vi "LoopSafe.vi"(6 "ModeChange Cluster":T1, 8 "error in (no error)":errorcluster, 11 "ModeCol in":refnum<class "ModeCol.lvclass">) -> (0 "error out":errorcluster, 3 "ModeCol out":refnum<class "ModeCol.lvclass">)   [LabVIEW 2013, in "ModeCol.lvclass"]
doc: "This VI check that there are no ramps between Loop-EndLoop pairs. It should be called only for \"Loop\" or \"EndLoop\" item tags."
uses:
  ModeCol.lvclass
  TypeDefs/ModeChange.ctl
  <vilib>/Utility/miscctls.llb/LVRowAndColumnTypeDef.ctl
  TypeDefs/TableHistory.ctl
  TypeDefs/TableArray.ctl
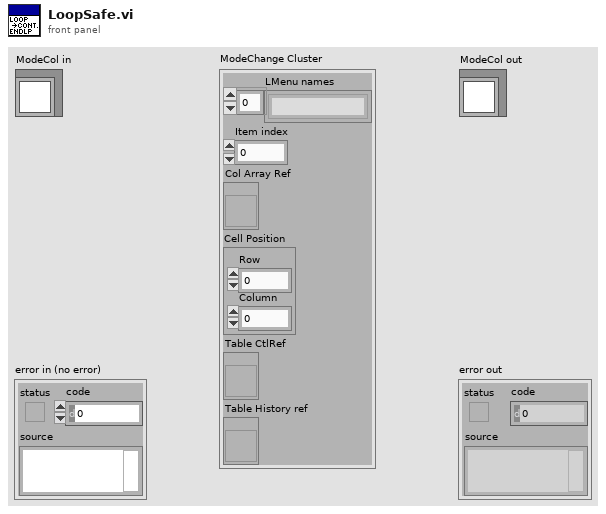
[diagram p1: front panel]
types:
  T1 = typedef "ModeChange.ctl" = cluster{"LMenu names":string[], "Item index":i32, "Col Array Ref":refnum<vi>, "Cell Position":T2, "Table CtlRef":refnum<vi>, "Table History ref":refnum<vi>}
  T2 = typedef "LVRowAndColumnTypeDef.ctl" = cluster{"Row":i32, "Column":i32}
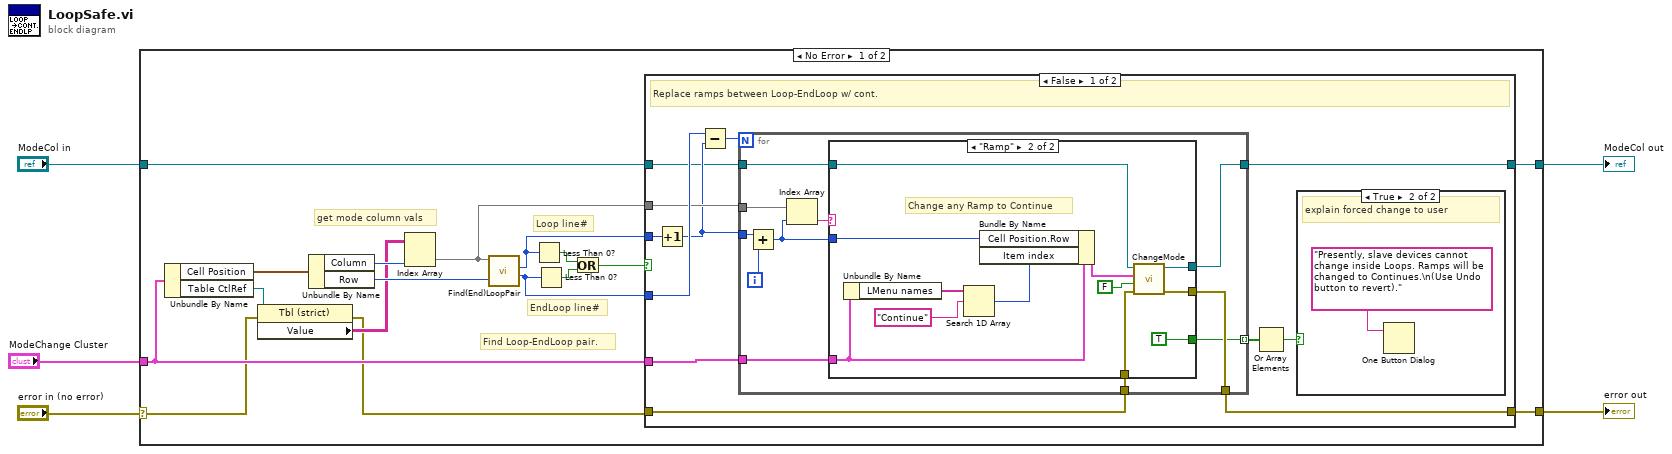
[diagram p0: block diagram]
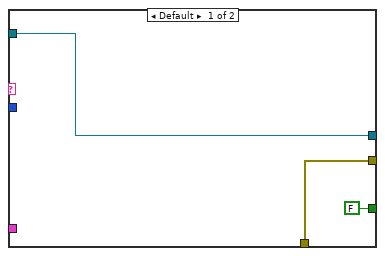
[diagram p3: hidden frame]
diagram:
  n1 = case shown="No Error" "error in (no error)" {
    selector: "error in (no error)" -> [w7 w65]
    tunnel: [w19 w65] -> w4
    tunnel: [w21 w64] -> w2
    tunnel: "ModeCol in" -> [w20 w64]
    tunnel: "ModeChange Cluster" -> [w10 _]
    frame No Error {
      # "Find Loop-EndLoop pair."
      # "EndLoop line#"
      # "Loop line#"
      # "get mode column vals"
      n2 = Unbundle By Name(w10) -> ("Cell Position"=w11:T2, "Table CtlRef"=w9:refnum<vi>)
      n3 = property class="Tbl (strict)"(reference=w9, error in=w7) -> (error out=w6:errorcluster, "Value"=w8:string[][])  [unwired: 1 out]
      n4 = Unbundle By Name(w11) -> ("Column"=w18:i32, "Row"=w22:i32)
      n5 = Index Array(array=w8, index (col)=w18) -> (element=w17:string[])  [unwired: 1 in]
      n6 = call "Find(End)LoopPair.vi"("(End)Loop index"=w22, "Mode Array"=w17) -> ("EndLoop index"=w12:i32, "Loop index"=w13:i32)  [unwired: 8 in]
      n7 = Less Than 0?(x=w13) -> (x < 0?=w15:bool)
      n8 = Less Than 0?(x=w12) -> (x < 0?=w16:bool)
      n9 = Or(x=w15, y=w16) -> (x .or. y?=w14:bool)
      n10 = case shown="False" w14 {
        tunnel: [w25 w63] -> w21
        tunnel: w20 -> [w26 w63]
        tunnel: [w33 w62] -> w19
        tunnel: w6 -> [w34 w62]
        tunnel: w13 -> [w31 _]
        tunnel: w12 -> [w30 _]
        tunnel: w17 -> [w28 _]
        tunnel: w10 -> [w32 _]
        frame False {
          # "Replace ramps between Loop-EndLoop w/ cont."
          n11 = Increment(x=w31) -> (x+1=w27:i32)
          n12 = Subtract(x=w30, y=w27) -> (x-y=w29:i32)
          n13 = for {
            N: w29 -> [_]
            tunnel: w34 -> [w46]
            tunnel: [w45] -> w33
            tunnel: w32 -> [w44]
            tunnel: w28 -> [w43]
            tunnel: w27 -> [w41]
            tunnel: w26 -> [w40]
            tunnel: [w39] -> w25
            tunnel: [w36] -> w24 mode=indexing
            i -> [w42]
            n14 = Add(x=w41, y=w42) -> (x+y=w37:i32)
            n15 = Index Array(array=w43, index=w37) -> (element=w38:string)
            n16 = case shown="\"Ramp\"" w38 {
              tunnel: w46 -> [w48 w59]
              tunnel: [w48 w60] -> w45
              tunnel: w44 -> [_ w55]
              tunnel: w40 -> [w49 w58]
              tunnel: [w49 w61] -> w39
              tunnel: w37 -> [_ w56]
              tunnel: [FALSE TRUE] -> w36
              frame Default {
              }
              frame "Ramp" {
                # "Change any Ramp to Continue"
                n17 = Unbundle By Name(w55) -> ("LMenu names"=w54:string[])
                n18 = Search 1D Array(1D array=w54, element="Continue") -> (index of element=w52:i32)  [unwired: 1 in]
                n19 = Bundle By Name(cluster=w55, "Cell Position.Row"=w56, "Item index"=w52) -> (w57:T1)
                n20 = call-dynamic "ChangeMode.vi"("error in (no error)"=w59, "Save to TblHist? (T)"=FALSE, "ModeChange Cluster"=w57, "ModeCol in"=w58) -> ("error out"=w60:errorcluster, "ModeCol out"=w61:refnum<class "ModeCol.lvclass">)  [unwired: 6 in]
              }
            }
          }
          n21 = Or Array Elements(Boolean array=w24) -> (logical OR=w23:bool)
          n22 = case shown="True" w23 {
            frame False {
            }
            frame True {
              # "explain forced change to user"
              n23 = One Button Dialog(message="Presently, slave devices cannot change inside Loops. Ramps will be changed to Continues.\n(Use Undo button to revert).") -> ()  [unwired: 1 in, 1 out]
            }
          }
        }
        frame True {
          # "do nothing if either is negative"
        }
      }
    }
    frame Error {
    }
  }
  "error out" <- w4
  "ModeCol out" <- w2
